vi "Configure Absolute Measurement.vi"(0 "VISA resource name":refnum<visa-resource-name>, 1 "Channel (1)":i32=1, 2 "Port (1)":i32=1, 3 "Trace (1)":i32=1, 9 "Measurement Parameter (0:S11)":u16(ring) items=["S11", "S21", "S31", "S41", "S12", "S22", "S32", "S42", "S13", "S23", "S33", "S43", "S14", "S24", "S34", "S44", "A", "B", "C", "D", "R1", "R2", "R3", "R4", "AUX1", "AUX2", "TR", "T", "R"], 11 "error in (no error)":errorcluster) -> (4 "VISA resource name out":refnum<visa-resource-name>, 15 "error out":errorcluster)   [LabVIEW 2012, in "Tektronix TTR500 Series.lvlib"]
doc: "This VI configures absolute measurement of active channel."
uses:
  <instrlib>/Tektronix TTR500 Series/Tektronix TTR500 Series.lvlib
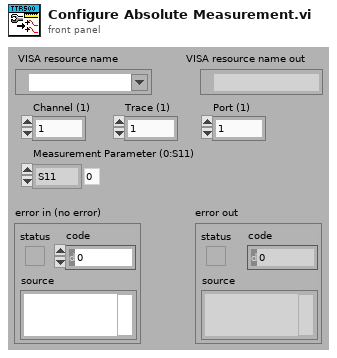
[diagram p1: front panel]
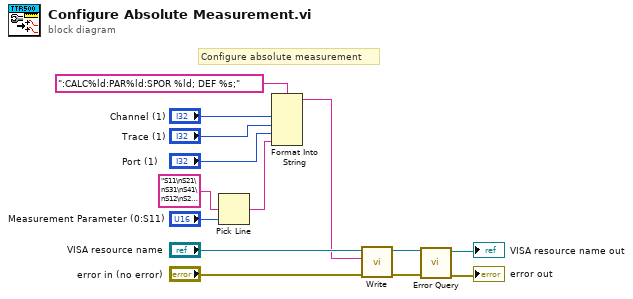
[diagram p0: block diagram]
diagram:
  # "Configure absolute measurement"
  n1 = Pick Line(multi-line string="S11\nS21\nS31\nS41\nS12\nS22\nS32\nS42\nS13\nS23\nS33\nS43\nS14\nS24\nS34\nS44\nA\nB\nC\nD\nR1\nR2\nR3\nR4\nAUX1\nAUX2\nTR\nT\nR", line index="Measurement Parameter (0:S11)") -> (output string=w12:string)  [unwired: 1 in]
  n2 = Format Into String(format string=":CALC%ld:PAR%ld:SPOR %ld; DEF %s;", "Channel (1)", "Trace (1)", "Port (1)", w12) -> (resulting string=w1:string)  [unwired: 2 in, 1 out]
  n3 = call <instrlib>:"Write.vi"("error in (no error)"="error in (no error)", "String ()"=w1, "VISA resource name"="VISA resource name") -> ("error out"=w6:errorcluster, "VISA resource name out"=w7:refnum<visa-resource-name>)  [unwired: 6 in, 1 out]
  n4 = call <instrlib>:"Error Query.vi"("error in (no error)"=w6, "VISA resource name"=w7) -> ("error out"=→"error out":errorcluster, "VISA resource name out"=→"VISA resource name out":refnum<visa-resource-name>)  [unwired: 6 in, 2 out]
